vi "StopPeriodicTrigger.vi"(8 "error in (no error)":errorcluster, 11 "TriggerID":u32) -> (0 "error out":errorcluster)   [LabVIEW 2020, in "PeriodicTrigger.lvlib"]
uses:
  PeriodicTrigger.lvlib
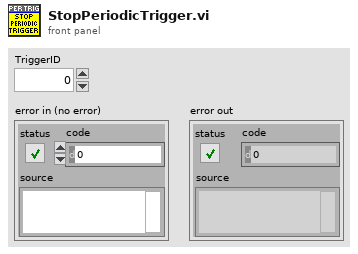
[diagram p1: front panel]
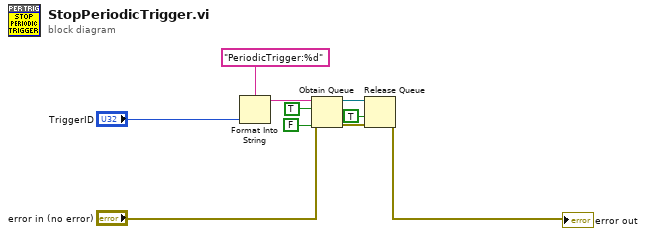
[diagram p0: block diagram]
diagram:
  n1 = Format Into String(format string="PeriodicTrigger:%d", "TriggerID") -> (resulting string=w10:string)  [unwired: 2 in, 1 out]
  n2 = Obtain Queue(name (unnamed)=w10, element data type=TRUE, create if not found? (T)=FALSE, error in (no error)="error in (no error)") -> (queue out=w6:refnum<queue>, error out=w5:errorcluster)  [unwired: 1 in, 1 out]
  n3 = Release Queue(queue=w6, force destroy? (F)=TRUE, error in (no error)=w5) -> (error out=→"error out":errorcluster)  [unwired: 2 out]
